vi "client.vi"() -> ()   [LabVIEW 2016]
panel:
  out "Data Recver":bool[](array[boolean])
  in  "stop 2":bool
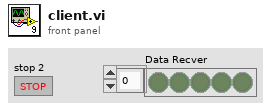
[diagram p1: front panel]
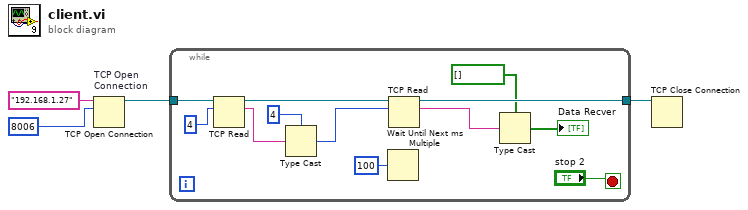
[diagram p0: block diagram]
diagram:
  n1 = TCP Open Connection "TCP Open \nConnection"(address="192.168.1.27", remote port or service name=u16 8006) -> (connection ID=w4:refnum<k5>)  [unwired: 3 in, 1 out]
  n2 = while {
    tunnel: w4 -> [w16]
    tunnel: [w14] -> w3
    stop <- "stop 2" stop-if-true
    n3 = TCP Read(connection ID=w16, bytes to read=4) -> (connection ID out=w15:refnum<k5>, data out=w11:string)  [unwired: 3 in, 1 out]
    n4 = Type Cast(type=4 ("bytes to read"), x=w11) -> (*(type *) &x=w10:i32)
    n5 = Wait Until Next ms Multiple(millisecond multiple=u32 100) -> ()  [unwired: 1 out]
    n6 = TCP Read(connection ID=w15, bytes to read=w10) -> (connection ID out=w14:refnum<k5>, data out=w9:string)  [unwired: 3 in, 1 out]
    n7 = Type Cast(type=bool[] [] ("Dato array"), x=w9) -> (*(type *) &x=→"Data Recver":bool[])
  }
  n8 = TCP Close Connection(connection ID=w3) -> ()  [unwired: 2 in, 2 out]
